vi "ShiftRegisters.vi"() -> ()   [LabVIEW 2025]
panel:
  in  "stop":bool
  out "X(i-3)":dbl
  out "X(i-2)":dbl
  out "X(i-1)":dbl
  out "X(i)":dbl
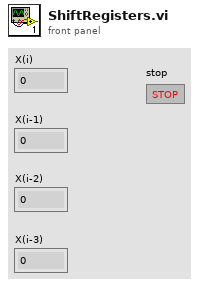
[diagram p1: front panel]
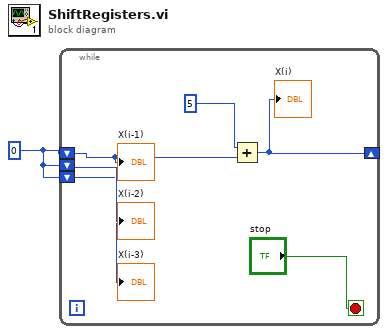
[diagram p0: block diagram]
diagram:
  w1 = 0
  n1 = while {
    shift-right: [w5] -> _
    shift-left: w1 -> [w2]
    shift-left: w1 -> [w4]
    shift-left: w1 -> [w3]
    stop <- "stop" stop-if-true
    n2 = Add(x=5, y=w2) -> (x+y=w5:i32)
    "X(i)" <- w5
    "X(i-1)" <- w2
    "X(i-2)" <- w4
    "X(i-3)" <- w3
  }
